vi "Load Create CFG File.vi"(8 "error in":errorcluster, 11 "Config in":refnum<class "Config.lvclass">) -> (0 "error out":errorcluster, 3 "Config out":refnum<class "Config.lvclass">)   [LabVIEW 2023, in "Config.lvlib" / "Config.lvclass"]
doc: "Load config.ini file path. If the file path is not found, create the file at the application root directory (which is the starting point for the recursive search)."
uses:
  Config.lvclass
  Config.lvclass/Config.ctl
  <vilib>/Utility/config.llb/NI_LVConfig.lvlib
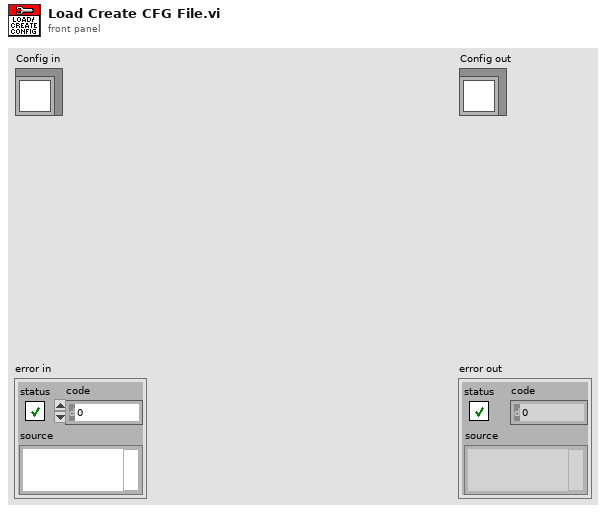
[diagram p1: front panel]
types:
  T1 = typedef "NI_LVConfig.lvlib/Config Data RefNum.ctl" = refnum<k1>
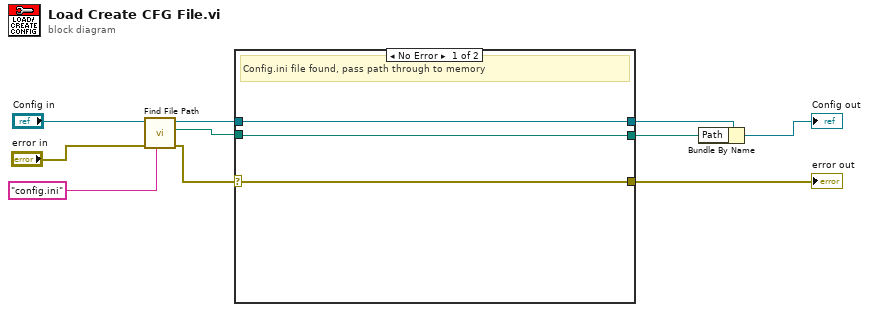
[diagram p0: block diagram]
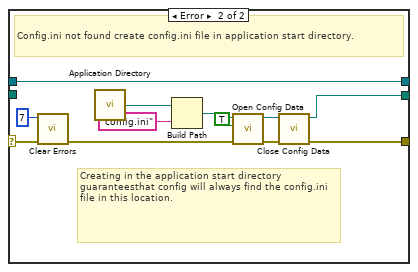
[diagram p2: hidden frame]
diagram:
  n1 = call "Find File Path.vi"("File Name\nwith extension"="config.ini" ("File Name\nwith extension"), "error in"="error in", "Config in"="Config in") -> ("error out"=w8:errorcluster, "File Path Control"=w6:path, "Config out"=w7:refnum<class "Config.lvclass">)  [unwired: 6 in]
  n2 = case shown="No Error" w8 {
    selector: w8 -> [w11 w16]
    tunnel: w7 -> [w13 w25]
    tunnel: w6 -> [w12 _]
    tunnel: [w13 w25] -> w5
    tunnel: [w12 w21] -> w3
    tunnel: [w11 w20] -> w2
    frame No Error {
      # "Config.ini file found, pass path through to memory"
    }
    frame Error {
      # "Creating in the application start directory guaranteesthat config will always find the config.ini file in this location."
      # "Config.ini not found create config.ini file in application start directory."
      n3 = call <vilib>:"Clear Errors.vi"("error in (no error)"=w16, "specific error code to clear (0: all)"=7) -> ("error out"=w14:errorcluster)  [unwired: 4 in, 1 out]
      n4 = call <vilib>:"Application Directory.vi"() -> ("Application Directory"=w24:path)
      n5 = Build Path(base path=w24, name or relative path="config.ini") -> (appended path=w18:path)
      n6 = call <vilib>:"Open Config Data.vi"("error in (no error)"=w14, "create file if necessary (T)"=TRUE, "configuration file path"=w18) -> ("error out"=w19:errorcluster, "refnum"=w22:T1)  [unwired: 6 in, 1 out]
      n7 = call <vilib>:"Close Config Data.vi"("error in (no error)"=w19, "refnum"=w22) -> ("error out"=w20:errorcluster, "file path"=w21:path)  [unwired: 8 in]
    }
  }
  "error out" <- w2
  n8 = Bundle By Name(cluster=w5, "Path"=w3) -> (→"Config out":refnum<class "Config.lvclass">)
